vi "test_shortest.vi"() -> ()   [LabVIEW 2019]
panel:
  out "forward?":bool
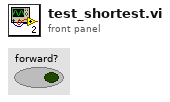
[diagram p1: front panel]
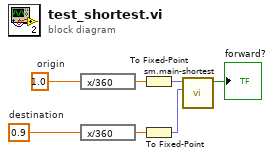
[diagram p0: block diagram]
diagram:
  w7 = 0.9  # destination
  w6 = 1.0  # origin
  n1 = expression code="x/360"(w6) -> (w5:dbl)
  n2 = expression code="x/360"(w7) -> (w4:dbl)
  n3 = To Fixed-Point(number=w5) -> (fixed-point=w3:fxp<+/-,32,2>)  [unwired: 1 in]
  n4 = To Fixed-Point(number=w4) -> (fixed-point=w2:fxp<+/-,32,2>)  [unwired: 1 in]
  n5 = call "sm.main-shortest.vi"("destination"=w2, "origin"=w3) -> ("forward?"=→"forward?":bool)  [unwired: 9 in]
